vi "TS Value.vi"(6 "Start Pressed":bool, 10 "NOK2":refnum<vi>, 11 "NOK1":refnum<vi>) -> (0 "Fix ID":string, 1 "Tool ID":string, 3 "Value":bool[](array[boolean]))   [LabVIEW 2023, in "GUI.lvlib"]
uses:
  GUI.lvlib
  <vilib>/DAQmx/read.llb/DAQmx Read (Digital 1D Bool NChan 1Samp 1Line).vi
  Global/Global TS.vi
  Global/Global LV.vi
  <vilib>/DAQmx/miscellaneous.llb/DAQmx Fill In Error Info.vi
panel:
  out "SCI Enable":bool
  out "HTTP Enable":bool
  out "MES Enable":bool
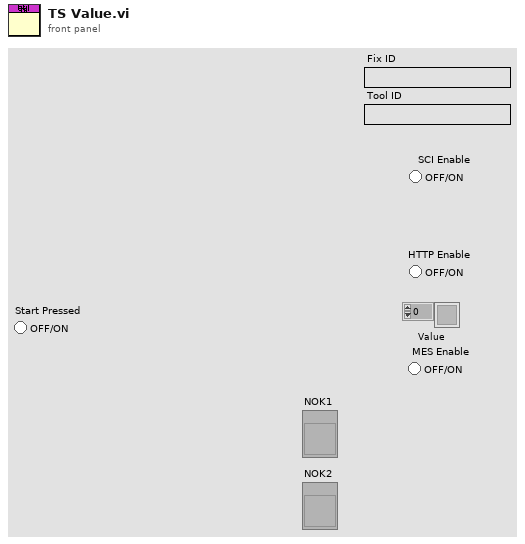
[diagram p1: front panel]
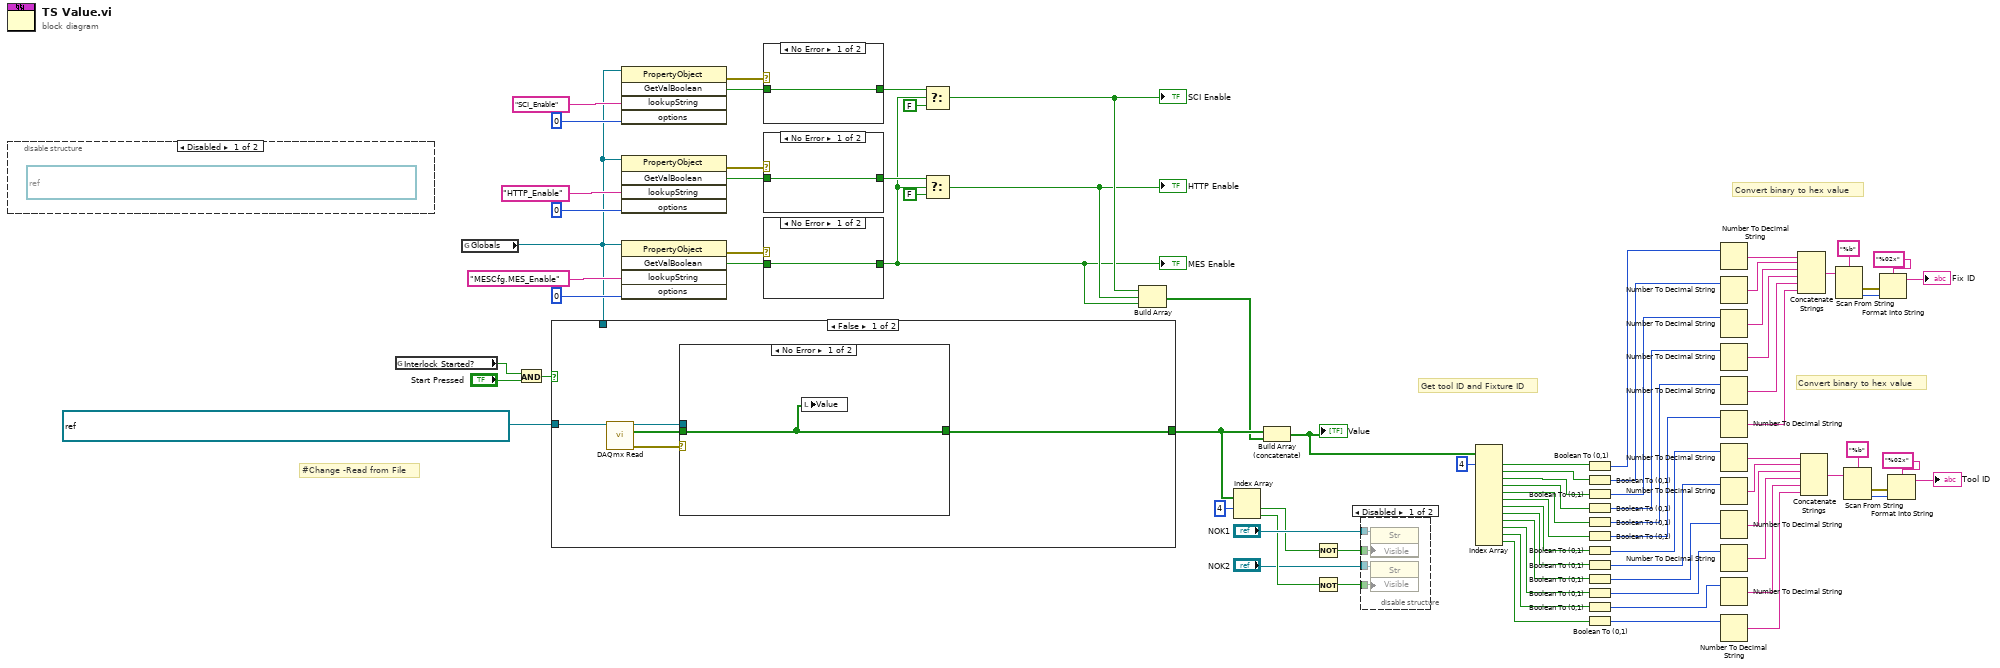
[diagram p0: block diagram]
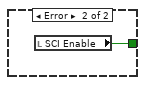
[diagram p4: hidden frame]
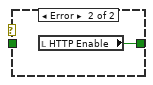
[diagram p5: hidden frame]
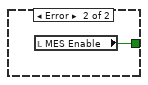
[diagram p6: hidden frame]
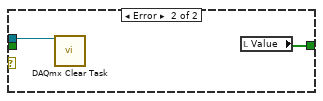
[diagram p7: hidden frame]
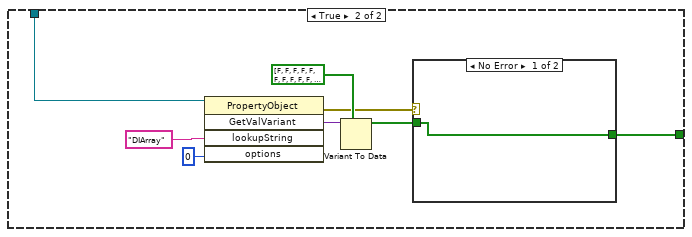
[diagram p8: hidden frame]
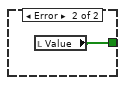
[diagram p9: hidden frame]
diagram:
  # "Convert binary to hex value"
  # "Convert binary to hex value"
  # "Get tool ID and Fixture ID"
  # "#Change -Read from File"
  n1 = disable-structure shown="Disabled" {
    frame Disabled {
      (unwired) refnum<k21> "Emergency, Fail Circuit Red FB, NOKBin1FB, NOKBin2FB, FixtureID1:6, ToolID1:6, Solinoid Coil FB, Home Position Sensor, Engaged Position Sensor, " ("DAQmx Global Channel")
    }
    frame Enabled {
    }
  }
  n2 = global read "Global LV.vi" "Interlock Started?"() -> (w71:bool)
  n3 = global read "Global TS.vi" "Globals"() -> (w61:refnum<k7>)
  n4 = And(x=w71, y="Start Pressed") -> (x .and. y?=w72:bool)
  n5 = case shown="False" w72 {
    tunnel: refnum<k21> "Emergency, Fail Circuit Red FB, NOKBin1FB, NOKBin2FB, FixtureID1:6, ToolID1:6, Solinoid Coil FB, Di-engage Position Sensor, Engaged Position Sensor, Home Position Sensor," ("DAQmx Global Channel") -> [w88 _]
    tunnel: [w87 w99] -> w56
    tunnel: w61 -> [_ w98]
    frame False {
      n6 = call-poly <vilib>:"DAQmx Read.vi"("task/channels in"=w88) -> ("task out"=w84:refnum<k21>, "data"=w86:bool[], "error out"=w85:errorcluster)  [unwired: 12 in]
      n7 = case shown="No Error" w85 {
        tunnel: w86 -> [w89 _]
        tunnel: [w89 w91] -> w87
        tunnel: w84 -> [_ w90]
        frame No Error {
          n8 = local write "Value"(w89) -> ()
        }
        frame Error {
          n9 = call <vilib>:"DAQmx Clear Task.vi"("task in"=w90) -> ()  [unwired: 14 in, 1 out]
          n10 = local read "Value"() -> (w91:bool[])
        }
      }
    }
    frame True {
      n11 = invoke class="PropertyObject" method="GetValVariant"(reference=w98, "lookupString"="DIArray" ("Lookup String"), "options"=0) -> (error out=w93:errorcluster, "GetValVariant"=w96:variant)  [unwired: 2 in, 3 out]
      n12 = Variant To Data(type=bool[] [FALSE, FALSE, FALSE, FALSE, FALSE, FALSE, FALSE, FALSE, FALSE, FALSE, FALSE, FALSE, FALSE, FALSE, FALSE, FALSE, FALSE, FALSE, FALSE], Variant=w96) -> (data=w92:bool[])  [unwired: 1 in, 1 out]
      n13 = case shown="No Error" w93 {
        tunnel: w92 -> [w100 _]
        tunnel: [w100 w101] -> w99
        frame No Error {
        }
        frame Error {
          n14 = local read "Value"() -> (w101:bool[])
        }
      }
    }
  }
  n15 = invoke class="PropertyObject" method="GetValBoolean"(reference=w61, "lookupString"="SCI_Enable", "options"=0) -> (error out=w64:errorcluster, "GetValBoolean"=w63:bool)  [unwired: 2 in, 3 out]
  n16 = invoke class="PropertyObject" method="GetValBoolean"(reference=w61, "lookupString"="HTTP_Enable", "options"=0) -> (error out=w67:errorcluster, "GetValBoolean"=w68:bool)  [unwired: 2 in, 3 out]
  n17 = invoke class="PropertyObject" method="GetValBoolean"(reference=w61, "lookupString"="MESCfg.MES_Enable", "options"=0) -> (error out=w75:errorcluster, "GetValBoolean"=w74:bool)  [unwired: 2 in, 3 out]
  n18 = case shown="No Error" w64 {
    tunnel: w63 -> [w102 _]
    tunnel: [w102 w103] -> w58
    frame No Error {
    }
    frame Error {
      n19 = local read "SCI Enable"() -> (w103:bool)
    }
  }
  n20 = case shown="No Error" w67 {
    tunnel: w68 -> [w104 _]
    tunnel: [w104 w105] -> w60
    frame No Error {
    }
    frame Error {
      n21 = local read "HTTP Enable"() -> (w105:bool)
    }
  }
  n22 = case shown="No Error" w75 {
    tunnel: w74 -> [w106 _]
    tunnel: [w106 w107] -> w53
    frame No Error {
    }
    frame Error {
      n23 = local read "MES Enable"() -> (w107:bool)
    }
  }
  "MES Enable" <- w53
  n24 = Select(t=w58, s=w53, f=FALSE) -> (s? t:f=w55:bool)
  "SCI Enable" <- w55
  n25 = Select(t=w60, s=w53, f=FALSE) -> (s? t:f=w54:bool)
  "HTTP Enable" <- w54
  n26 = Build Array(w55, w54, w53) -> (w51:bool[])
  n27 = Index Array(array=w56, index #1=4 ("index")) -> (element #1=w81:bool, element #2=w80:bool)  [unwired: 1 in]
  n28 = Build Array (concatenate)(w56, w51) -> (w50:bool[])
  "Value" <- w50
  n29 = Not(x=w81) -> (.not. x?=w78:bool)
  n30 = Not(x=w80) -> (.not. x?=w77:bool)
  n31 = disable-structure shown="Disabled" {
    disable-tunnel: "NOK1" -> [w111 _]
    disable-tunnel: "NOK2" -> [w110 _]
    disable-tunnel: w78 -> [w109 _]
    disable-tunnel: w77 -> [w108 _]
    frame Disabled {
      n32 = property class="Str"(reference=w111, "Visible"=w109) -> ()  [unwired: 1 in, 2 out]
      n33 = property class="Str"(reference=w110, "Visible"=w108) -> ()  [unwired: 1 in, 2 out]
    }
    frame Enabled {
    }
  }
  n34 = Index Array(array=w50, index #1=4 ("index")) -> (element #1=w48:bool, element #2=w47:bool, element #3=w46:bool, element #4=w45:bool, element #5=w44:bool, element #6=w43:bool, element #7=w42:bool, element #8=w41:bool, element #9=w40:bool, element #10=w39:bool, element #11=w38:bool, element #12=w37:bool)  [unwired: 11 in]
  n35 = Boolean To (0,1)(Boolean=w48) -> (0, 1=w36:i16)
  n36 = Boolean To (0,1)(Boolean=w47) -> (0, 1=w35:i16)
  n37 = Boolean To (0,1)(Boolean=w46) -> (0, 1=w34:i16)
  n38 = Boolean To (0,1)(Boolean=w45) -> (0, 1=w25:i16)
  n39 = Boolean To (0,1)(Boolean=w44) -> (0, 1=w33:i16)
  n40 = Boolean To (0,1)(Boolean=w43) -> (0, 1=w32:i16)
  n41 = Boolean To (0,1)(Boolean=w42) -> (0, 1=w31:i16)
  n42 = Boolean To (0,1)(Boolean=w41) -> (0, 1=w30:i16)
  n43 = Boolean To (0,1)(Boolean=w40) -> (0, 1=w29:i16)
  n44 = Boolean To (0,1)(Boolean=w39) -> (0, 1=w28:i16)
  n45 = Boolean To (0,1)(Boolean=w38) -> (0, 1=w27:i16)
  n46 = Boolean To (0,1)(Boolean=w37) -> (0, 1=w26:i16)
  n47 = Number To Decimal String(number=w36) -> (decimal integer string=w24:string)  [unwired: 1 in]
  n48 = Number To Decimal String(number=w35) -> (decimal integer string=w23:string)  [unwired: 1 in]
  n49 = Number To Decimal String(number=w34) -> (decimal integer string=w22:string)  [unwired: 1 in]
  n50 = Number To Decimal String(number=w25) -> (decimal integer string=w21:string)  [unwired: 1 in]
  n51 = Number To Decimal String(number=w33) -> (decimal integer string=w20:string)  [unwired: 1 in]
  n52 = Number To Decimal String(number=w32) -> (decimal integer string=w19:string)  [unwired: 1 in]
  n53 = Number To Decimal String(number=w31) -> (decimal integer string=w18:string)  [unwired: 1 in]
  n54 = Number To Decimal String(number=w30) -> (decimal integer string=w17:string)  [unwired: 1 in]
  n55 = Number To Decimal String(number=w29) -> (decimal integer string=w16:string)  [unwired: 1 in]
  n56 = Number To Decimal String(number=w28) -> (decimal integer string=w15:string)  [unwired: 1 in]
  n57 = Number To Decimal String(number=w27) -> (decimal integer string=w14:string)  [unwired: 1 in]
  n58 = Number To Decimal String(number=w26) -> (decimal integer string=w13:string)  [unwired: 1 in]
  n59 = Concatenate Strings(w24, w23, w22, w21, w20, w19) -> (w1:string)
  n60 = Concatenate Strings(w18, w17, w16, w15, w14, w13) -> (w2:string)
  n61 = Scan From String(format string="%b", input string=w1) -> (error out=w11:errorcluster, output 1=w12:i32)  [unwired: 3 in, 2 out]
  n62 = Scan From String(format string="%b", input string=w2) -> (error out=w8:errorcluster, output 1=w3:i32)  [unwired: 3 in, 2 out]
  n63 = Format Into String(format string="%02x", error in=w11, w12) -> (resulting string=→"Fix ID":string)  [unwired: 1 in, 1 out]
  n64 = Format Into String(format string="%02x", error in=w8, w3) -> (resulting string=→"Tool ID":string)  [unwired: 1 in, 1 out]
